vi "readMotorEncoder (SubVI).vi"(6 "reset Encoder":bool, 7 "Motor ID":T1, 8 "Error In":errorcluster, 11 "TitanQuad in":refnum<class "TitanQuad.lvclass">) -> (0 "Error Out":errorcluster, 2 "Enc (deg)":dbl, 3 "TitanQuad out":refnum<class "TitanQuad.lvclass">)   [LabVIEW 2020]
uses:
  <vilib>/CISH Robotics/L4VMX TitanQuad/Motor ID.ctl
  <vilib>/CISH Robotics/L4VMX TitanQuad/TitanQuad.lvclass
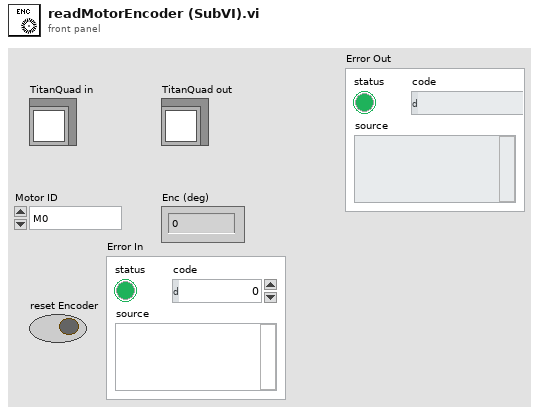
[diagram p1: front panel]
types:
  T1 = typedef "TitanQuad.lvlib/TitanQuad.lvclass/Motor ID.ctl" = enum16{"M0", "M1", "M2", "M3"}
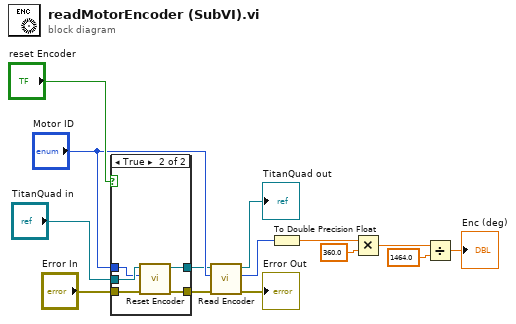
[diagram p0: block diagram]
diagram:
  n1 = case shown="True" "reset Encoder" {
    tunnel: "TitanQuad in" -> [w16 w21]
    tunnel: [w16 w20] -> w12
    tunnel: "Motor ID" -> [_ w19]
    tunnel: "Error In" -> [w15 w18]
    tunnel: [w15 w17] -> w2
    frame False {
    }
    frame True {
      n2 = call <vilib>:"Reset Encoder.vi"("Error In"=w18, "Motor ID"=w19, "TitanQuad Object"=w21) -> ("Error Out"=w17:errorcluster, "TitanQuad Object"=w20:refnum<class "TitanQuad.lvclass">)  [unwired: 7 in]
    }
  }
  n3 = call <vilib>:"Read Encoder.vi"("Error In"=w2, "Motor ID"="Motor ID", "TitanQuad Object"=w12) -> ("Error Out"=→"Error Out":errorcluster, "Counter Value"=w6:i32, "TitanQuad Object"=→"TitanQuad out":refnum<class "TitanQuad.lvclass">)  [unwired: 6 in]
  n4 = To Double Precision Float(number=w6) -> (double precision float=w7:dbl)
  n5 = Multiply(x=w7, y=360.0) -> (x*y=w5:dbl)
  n6 = Divide(x=w5, y=1464.0) -> (x/y=→"Enc (deg)":dbl)
